vi "Write ForgetFactor.vi"(8 "error in (no error)":errorcluster, 10 "ForgetFactor":dbl, 11 "Probabilistic_OccupancyGrid in":refnum<class "Probabilistic_OccupancyGrid.lvclass">) -> (0 "error out":errorcluster, 3 "Probabilistic_OccupancyGrid out":refnum<class "Probabilistic_OccupancyGrid.lvclass">)   [LabVIEW 2017, in "Probabilistic_OccupancyGrid.lvclass"]
uses:
  Probabilistic_OccupancyGrid.lvclass
  Probabilistic_OccupancyGrid.lvclass/Probabilistic_OccupancyGrid.ctl
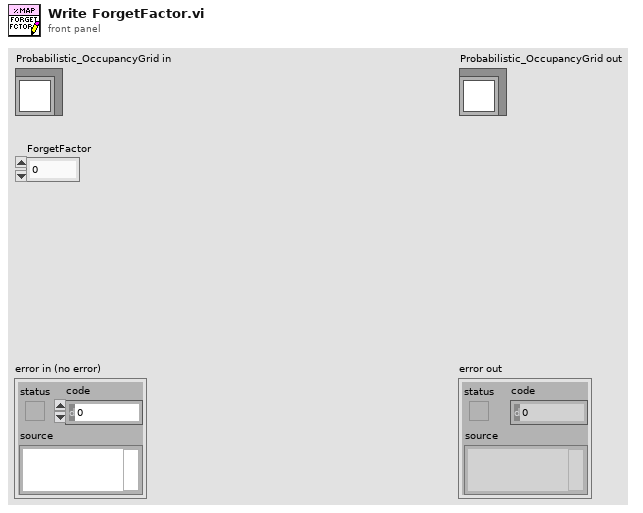
[diagram p1: front panel]
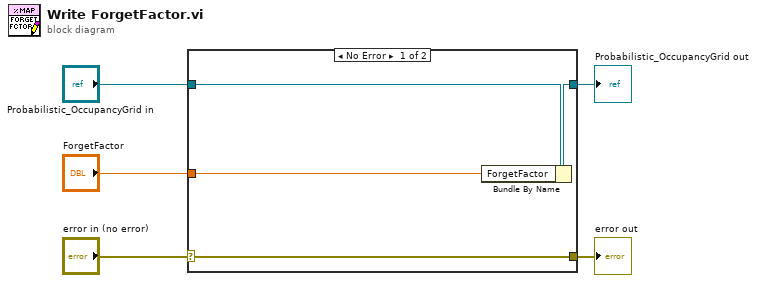
[diagram p0: block diagram]
diagram:
  n1 = case shown="No Error" "error in (no error)" {
    selector: "error in (no error)" -> [w9 w10]
    tunnel: [w9 w10] -> w4
    tunnel: [w7 w11] -> w2
    tunnel: "Probabilistic_OccupancyGrid in" -> [w8 w11]
    tunnel: "ForgetFactor" -> [w6 _]
    frame No Error {
      n2 = Bundle By Name(cluster=w8, "ForgetFactor"=w6) -> (w7:refnum<class "Probabilistic_OccupancyGrid.lvclass">)
    }
    frame Error {
    }
  }
  "error out" <- w4
  "Probabilistic_OccupancyGrid out" <- w2
